vi "Conveyer Belt Set.vi"(1 "Conveyer Belt Information In":T1) -> (0 "Conveyer Belt Information Out":T1)   [LabVIEW 2012]
uses:
  <vilib>/Rock Robotics/WPI/DriverStation/WPI_DriverStationRobotMode2.ctl
  Extras/Global Data.vi
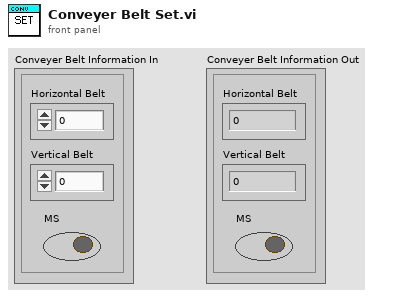
[diagram p1: front panel]
types:
  T1 = cluster{"Horizontal Belt":dbl, "Vertical Belt":dbl, "MS":bool}
  T2 = typedef "WPI_DriverStationRobotMode2.ctl" = enum16{"Autonomous Disabled", "Autonomous Enabled", "Teleop Disabled", "Teleop Enabled", "Timeout", "Finish", "Test Disabled", "Test Enabled"}
  T3 = typedef "WPI_RelayValue.ctl" = enum16{"Off", "On", "Forward", "Reverse"}
  T4 = typedef "WPI_RelayDevRef.ctl" = cluster{"DevStatus":errorcluster, "Relay Channel":T5, "Digital Module":T6, "Relay Direction":T7}
  T5 = typedef "FPGA_DIORelayChannel.ctl" = enum8{"Relay 1", "Relay 2", "Relay 3", "Relay 4", "Relay 5", "Relay 6", "Relay 7", "Relay 8", "Invalid"}
  T6 = typedef "FPGA_TypedefDigitalModule.ctl" = enum16{"Digital Module 1", "Digital Module 2"}
  T7 = typedef "WPI_RelayDirection.ctl" = enum16{"Both directions", "Forward only", "Reverse only"}
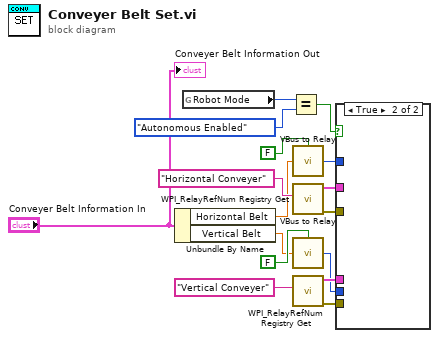
[diagram p0: block diagram]
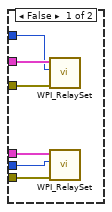
[diagram p2: hidden frame]
diagram:
  n1 = Unbundle By Name("Conveyer Belt Information In") -> ("Horizontal Belt"=w14:dbl, "Vertical Belt"=w11:dbl)
  n2 = global read "Global Data.vi" "Robot Mode"() -> (w7:T2)
  n3 = Equal?(x=w7, y=WPI_DriverStationRobotMode2."Autonomous Enabled" ("Robot Mode")) -> (x = y?=w9:bool)
  n4 = call "VBus to Relay.vi"("Invert Relay? (F)"=FALSE, "Motor VBus"=w14) -> ("RelayValue"=w4:T3)  [unwired: 2 in]
  n5 = call <vilib>:"WPI_RelayRefNum Registry Get.vi"("refnum name"="Horizontal Conveyer") -> ("error out"=w5:errorcluster, "RelayDevRef"=w6:T4)  [unwired: 9 in]
  n6 = call "VBus to Relay.vi"("Invert Relay? (F)"=FALSE, "Motor VBus"=w11) -> ("RelayValue"=w2:T3)  [unwired: 2 in]
  n7 = call <vilib>:"WPI_RelayRefNum Registry Get.vi"("refnum name"="Vertical Conveyer") -> ("error out"=w1:errorcluster, "RelayDevRef"=w3:T4)  [unwired: 9 in]
  n8 = case shown="True" w9 {
    tunnel: w6 -> [w22 _]
    tunnel: w5 -> [w21 _]
    tunnel: w4 -> [w20 _]
    tunnel: w3 -> [w19 _]
    tunnel: w2 -> [w18 _]
    tunnel: w1 -> [w17 _]
    frame False {
      n9 = call <vilib>:"WPI_RelaySet.vi"("error in (no error)"=w21, "RelayValue"=w20, "RelayDevRef"=w22) -> ()  [unwired: 7 in, 2 out]
      n10 = call <vilib>:"WPI_RelaySet.vi"("error in (no error)"=w17, "RelayValue"=w18, "RelayDevRef"=w19) -> ()  [unwired: 7 in, 2 out]
    }
    frame True {
    }
  }
  "Conveyer Belt Information Out" <- "Conveyer Belt Information In"
